vi "icListen 2 Saving.vi"() -> ()   [LabVIEW 2020, in "PAM Library.lvlib"]
uses:
  PAM Library.lvlib
panel:
  in  "icListen 2 Saving":bool
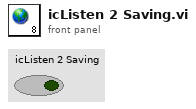
[diagram p1: front panel]
diagram:
